vi "Key - String Read.vi"(8 "error in (no error)":errorcluster, 9 "New String Ref":refnum<vi>, 10 "Original String Ref":refnum<vi>, 11 "Refnum in":T1) -> (0 "error out":errorcluster, 2 "spreadsheet string":string, 3 "Refnum out":T1)   [LabVIEW 2013]
uses:
  <vilib>/Utility/config.llb/Config Data RefNum.ctl
  <vilib>/Utility/config.llb/Read Key (String).vi
  <vilib>/Utility/config.llb/NI_LVConfig.lvlib
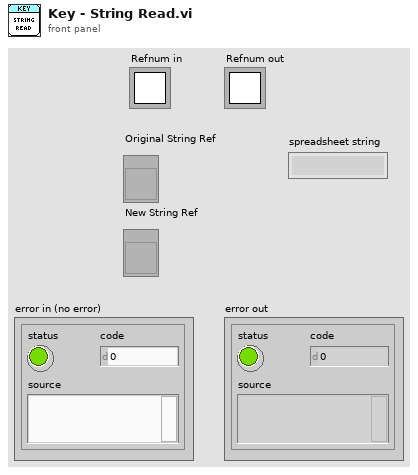
[diagram p1: front panel]
types:
  T1 = typedef "NI_LVConfig.lvlib/Config Data RefNum.ctl" = refnum<k1>
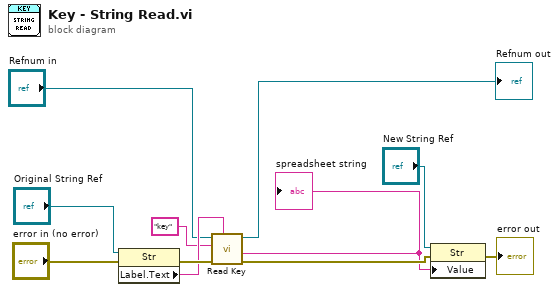
[diagram p0: block diagram]
diagram:
  n1 = property class="Str"(reference="Original String Ref", error in="error in (no error)") -> (error out=w10:errorcluster, "Label.Text"=w8:string)  [unwired: 1 out]
  n2 = call-poly <vilib>:"Read Key.vi"("section"=w8, "error in (no error)"=w10, "key"="key" ("section"), "refnum"="Refnum in") -> ("error out"=w11:errorcluster, "value"=w2:string, "refnum out"=→"Refnum out":T1)  [unwired: 4 in, 1 out]
  "spreadsheet string" <- w2
  n3 = property class="Str"(reference="New String Ref", error in=w11, "Value"=w2) -> (error out=→"error out":errorcluster)  [unwired: 1 out]
